vi "Save Test Data.vi"(8 "error in (no error)":errorcluster, 10 "Test Data":string[](array[string]), 11 "Access in":refnum<class "Access.lvclass">) -> (0 "error out":errorcluster, 3 "Access out":refnum<class "Access.lvclass">)   [LabVIEW 2021, in "Database.lvlib" / "Access.lvclass"]
uses:
  Access.lvclass
  Access.lvclass/Access.ctl
  <vilib>/addons/database/NI_Database_API.lvlib
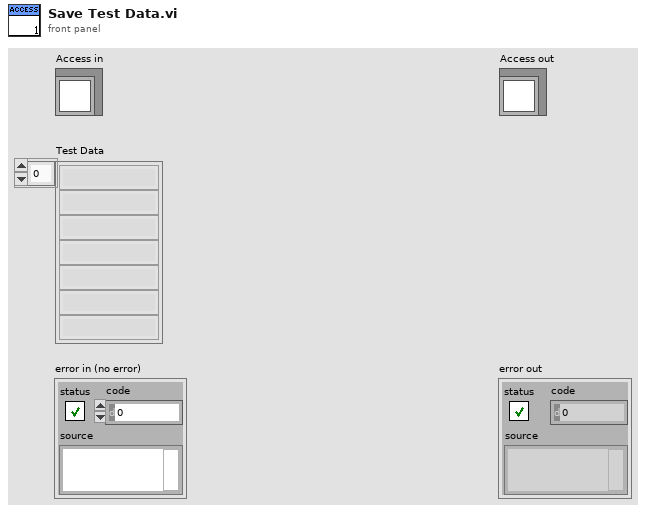
[diagram p1: front panel]
types:
  T1 = typedef "Database.lvlib/DB.lvclass/Table_info.ctl" = cluster{"Authentication":string, "Instr_Configuration":string, "Recipe":string, "Test_data":string}
  T2 = typedef "NI_Database_API.lvlib/Conn ObjectReference.ctl" = refnum<k1>
  T3 = cluster{"[0]":string, "[1]":string, "[2]":string, "[3]":string, "[4]":string, "[5]":string}
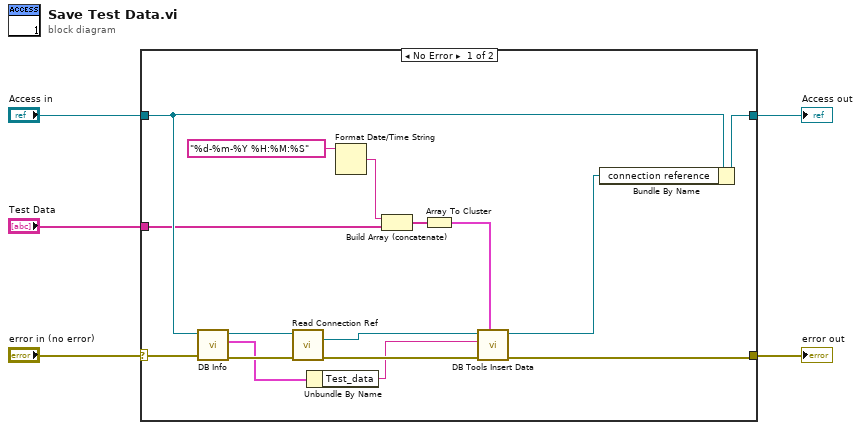
[diagram p0: block diagram]
diagram:
  n1 = case shown="No Error" "error in (no error)" {
    selector: "error in (no error)" -> [w21 w23]
    tunnel: "Access in" -> [w20 w22]
    tunnel: [w14 w22] -> w3
    tunnel: [w15 w23] -> w2
    tunnel: "Test Data" -> [w9 _]
    frame No Error {
      n2 = call-dynamic "DB Info.vi"("error in (no error)"=w21, "Access in"=w20) -> ("error out"=w19:errorcluster, "Table_info"=w11:T1, "Access out"=w18:refnum<class "Access.lvclass">)  [unwired: 6 in, 1 out]
      n3 = call-dynamic "Read Connection Ref.vi"("error in (no error)"=w19, "Access in"=w18) -> ("error out"=w16:errorcluster, "connection reference"=w12:T2)  [unwired: 7 in, 1 out]
      n4 = Unbundle By Name(w11) -> ("Test_data"=w10:string)
      n5 = Format Date/Time String(time format string (%c)="%d-%m-%Y %H:%M:%S") -> (date/time string=w8:string)  [unwired: 2 in]
      n6 = Build Array (concatenate)(w8, w9) -> (w7:string[])
      n7 = Array To Cluster(array=w7) -> (cluster=w6:T3)
      n8 = call <vilib>:"DB Tools Insert Data.vi"("data"=w6, "error in (no error)"=w16, "table"=w10, "connection reference"=w12) -> ("error out"=w15:errorcluster, "connection reference out"=w13:T2)  [unwired: 6 in]
      n9 = Bundle By Name(cluster=w20, "connection reference"=w13) -> (w14:refnum<class "Access.lvclass">)
    }
    frame Error {
    }
  }
  "error out" <- w2
  "Access out" <- w3
